vi "Add Point.vi"(8 "error in (no error)":errorcluster, 10 "3D Point":cluster{"X":sgl, "Y":sgl, "Z":sgl}, 11 "Trajectory Drawer in":refnum<class "Trajectory Drawer.lvclass">) -> (0 "error out":errorcluster, 3 "Trajectory Drawer out":refnum<class "Trajectory Drawer.lvclass">)   [LabVIEW 2014, in "Trajectory Drawer.lvclass"]
uses:
  Trajectory Drawer.lvclass
  <vilib>/Utility/miscctls.llb/LVRGBAColorTypeDef.ctl
  Trajectory Drawer.lvclass/Trajectory Drawer.ctl
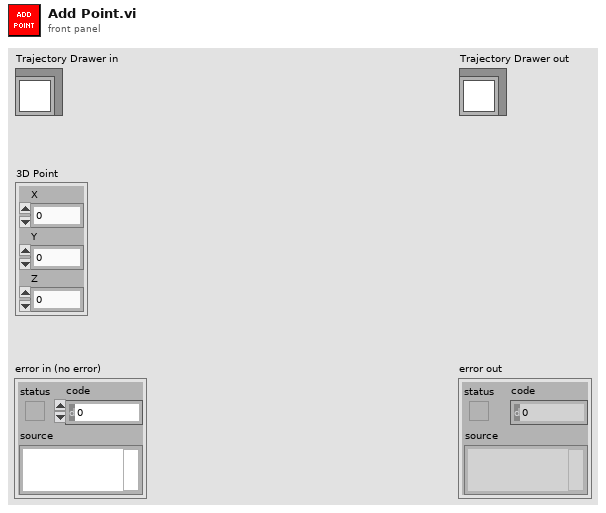
[diagram p1: front panel]
types:
  T1 = typedef "LVRGBAColorTypeDef.ctl" = cluster{"Red":sgl, "Green":sgl, "Blue":sgl, "Alpha":sgl}
  T2 = enum16{"Points", "Lines", "Line Strip", "Line Loop", "Triangles", "Triangle Strip", "Triangle Fan", "Quads", "Quad Strip", "Polygon"}
  T3 = enum16{"Overall", "Per Primitive", "Per Vertex", "Binding Off"}
  T4 = typedef "LV3DPointTypeDef.ctl" = cluster{"X":sgl, "Y":sgl, "Z":sgl}
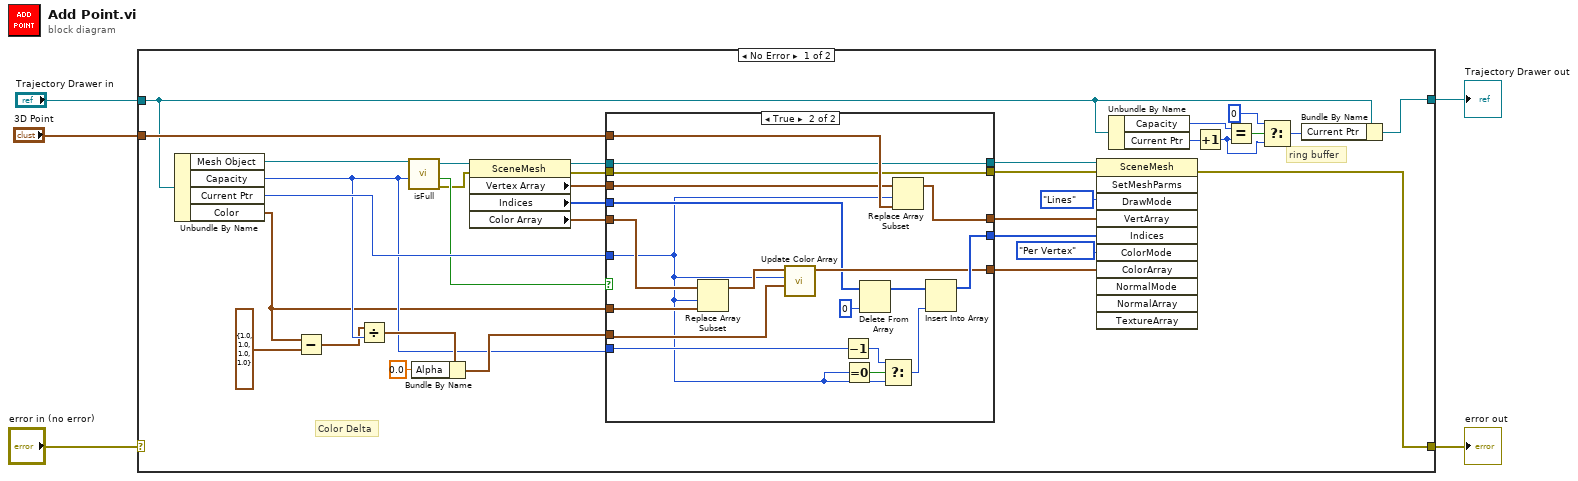
[diagram p0: block diagram]
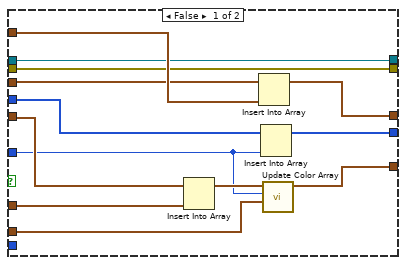
[diagram p2: hidden frame]
diagram:
  n1 = case shown="No Error" "error in (no error)" {
    selector: "error in (no error)" -> [_ w73]
    tunnel: [w13 w73] -> w4
    tunnel: [w30 w72] -> w3
    tunnel: "3D Point" -> [w38 _]
    tunnel: "Trajectory Drawer in" -> [w15 w72]
    frame No Error {
      # "ring buffer"
      # "Color Delta"
      n2 = Unbundle By Name(w15) -> ("Mesh Object"=w39:refnum<vi>, "Capacity"=w14:i32, "Current Ptr"=w37:i32, "Color"=w8:T1)
      n3 = Subtract(x=w8, y=T1 {"Red"=1.0, "Green"=1.0, "Blue"=1.0, "Alpha"=1.0} ("Color")) -> (x-y=w7:T1)
      n4 = Divide(x=w7, y=w14) -> (x/y=w28:T1)
      n5 = call "isFull.vi"("Capacity"=w14, "Object In"=w39) -> ("error out"=w11:errorcluster, "Full?"=w29:bool, "Mesh Ref"=w12:refnum<vi>)  [unwired: 7 in]
      n6 = Bundle By Name(cluster=w28, "Alpha"=0.0) -> (w27:T1)
      n7 = property class="SceneMesh"(reference=w12, error in=w11) -> (reference out=w16:refnum<vi>, error out=w20:errorcluster, "Vertex Array"=w19:T4[], "Indices"=w18:u32[], "Color Array"=w17:T1[])
      n8 = case shown="True" w29 {
        tunnel: w16 -> [w43 w58]
        tunnel: w38 -> [w52 w69]
        tunnel: w37 -> [w40 w53]
        tunnel: w14 -> [_ w63]
        tunnel: w8 -> [w49 w62]
        tunnel: w27 -> [w50 w70]
        tunnel: w20 -> [w42 w57]
        tunnel: [w43 w58] -> w25
        tunnel: [w42 w57] -> w24
        tunnel: [w47 w61] -> w23
        tunnel: [w48 w60] -> w22
        tunnel: [w46 w59] -> w21
        tunnel: w19 -> [w45 w56]
        tunnel: w18 -> [w41 w55]
        tunnel: w17 -> [w44 w54]
        frame False {
          n9 = Insert Into Array(array=w44, new element=w49) -> (w51:T1[])  [unwired: 1 in]
          n10 = Insert Into Array(array=w45, new element=w52) -> (w48:T4[])  [unwired: 1 in]
          n11 = Insert Into Array(array=w41, new element=w40) -> (w47:u32[])  [unwired: 1 in]
          n12 = call "Update Color Array.vi"("Color Delta"=w50, "Current Index"=w40, "Color Array"=w51) -> ("Updated Color"=w46:cluster{dbl, dbl, dbl, dbl}[])  [unwired: 8 in]
        }
        frame True {
          n13 = Replace Array Subset(array=w54, new element=w62, index=w53) -> (w71:T1[])
          n14 = call "Update Color Array.vi"("Color Delta"=w70, "Current Index"=w53, "Color Array"=w71) -> ("Updated Color"=w59:cluster{dbl, dbl, dbl, dbl}[])  [unwired: 8 in]
          n15 = Decrement(x=w63) -> (x-1=w67:i32)
          n16 = Equal To 0?(x=w53) -> (x = 0?=w68:bool)
          n17 = Delete From Array(array=w55, index=0) -> (array with subset deleted=w66:u32[])  [unwired: 1 in, 1 out]
          n18 = Select(t=w67, s=w68, f=w53) -> (s? t:f=w64:i32)
          n19 = Replace Array Subset(array=w56, new element=w69, index=w53) -> (w60:T4[])
          n20 = Insert Into Array(array=w66, new element=w64) -> (w61:u32[])  [unwired: 1 in]
        }
      }
      n21 = invoke class="SceneMesh" method="SetMeshParms"(reference=w25, error in=w24, "DrawMode"=T2."Lines" ("Draw Mode"), "VertArray"=w22, "Indices"=w23, "ColorMode"=T3."Per Vertex" ("Color Binding Mode"), "ColorArray"=w21) -> (error out=w13:errorcluster)  [unwired: 4 in, 10 out]
      n22 = Unbundle By Name(w15) -> ("Capacity"=w35:i32, "Current Ptr"=w36:i32)
      n23 = Increment(x=w36) -> (x+1=w32:i32)
      n24 = Equal?(x=w35, y=w32) -> (x = y?=w34:bool)
      n25 = Select(t=0, s=w34, f=w32) -> (s? t:f=w31:i32)
      n26 = Bundle By Name(cluster=w15, "Current Ptr"=w31) -> (w30:refnum<class "Trajectory Drawer.lvclass">)
    }
    frame Error {
    }
  }
  "error out" <- w4
  "Trajectory Drawer out" <- w3
